vi "Find All Uses.Bundlers.vi"(9 "Fully Qualified Array":string[](array[string]), 10 "dotted name":cluster{"dotted name":string[]}, 11 "VIs":refnum<vi>[](array[refnum])) -> (2 "bundle":refnum<vi>[](array[refnum]), 3 "named bundle":refnum<vi>[](array[refnum]))   [LabVIEW 2020]
uses:
  <vilib>/Utility/traverseref.llb/TRef TravTarget.ctl
  <vilib>/Utility/traverseref.llb/VI Scripting - Traverse.lvlib
  <vilib>/Utility/Data Type/NI_Data Type.lvlib
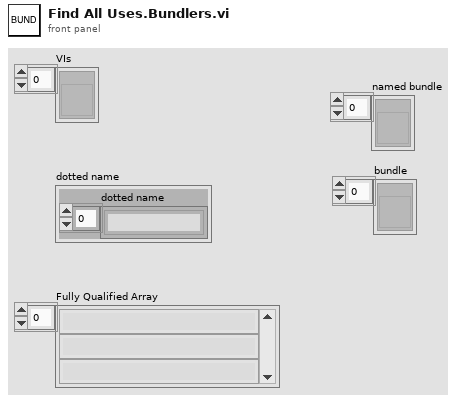
[diagram p1: front panel]
types:
  T1 = typedef "TRef TravTarget.ctl" = enum16{"FP", "BD", "Other"}
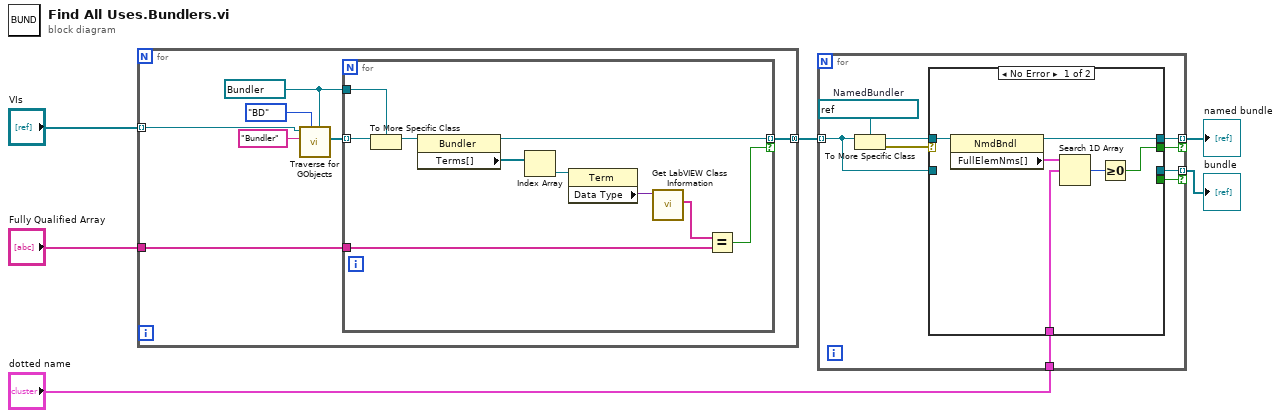
[diagram p0: block diagram]
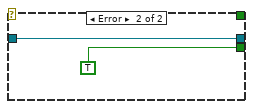
[diagram p2: hidden frame]
diagram:
  n1 = for {
    tunnel: "VIs" -> [w13] mode=indexing
    tunnel: [w8] -> w4 mode=concatenating
    tunnel: "Fully Qualified Array" -> [w7]
    w9 = refnum<vi> refnum ("Other Refnum")
    n2 = call <vilib>:"Traverse for GObjects.vi"("Other Refnum"=w9, "Traverse Target"=TRef_TravTarget."BD", "Class Name"="Bundler", "VI Refnum"=w13) -> ("References"=w10:refnum<vi>[])  [unwired: 4 in, 3 out]
    n3 = for {
      tunnel: w10 -> [w23] mode=indexing
      tunnel: w9 -> [w22]
      tunnel: [w20] -> w8 mode=indexing if=w14
      tunnel: w7 -> [w15]
      n4 = To More Specific Class(target class=w22, reference=w23) -> (specific class reference=w21:refnum<vi>)  [unwired: 1 in, 1 out]
      n5 = property class="Bundler"(reference=w21) -> (reference out=w20:refnum<vi>, "Terms[]"=w19:refnum<vi>[])  [unwired: 1 in, 1 out]
      n6 = Index Array(array=w19) -> (element=w18:refnum<vi>)  [unwired: 1 in]
      n7 = property class="Term"(reference=w18) -> ("Data Type"=w17:variant)  [unwired: 1 in, 2 out]
      n8 = call <vilib>:"Get LabVIEW Class Information.vi"("variant"=w17) -> ("qualified LabVIEW class name"=w16:string[])  [unwired: 8 in, 2 out]
      n9 = Equal?(x=w16, y=w15) -> (x = y?=w14:bool)
    }
  }
  n10 = for {
    tunnel: w4 -> [w29] mode=indexing
    tunnel: [w28] -> w2 mode=indexing if=w27
    tunnel: [w26] -> w3 mode=indexing if=w25
    tunnel: "dotted name" -> [w24]
    w32 = refnum<vi> refnum  # NamedBundler
    n11 = To More Specific Class(target class=w32, reference=w29) -> (specific class reference=w30:refnum<vi>, error out=w31:errorcluster)  [unwired: 1 in]
    n12 = case shown="No Error" w31 {
      tunnel: w30 -> [w36 _]
      tunnel: w29 -> [_ w40]
      tunnel: [_ w40] -> w28
      tunnel: [_ TRUE] -> w27
      tunnel: [w35 _] -> w26
      tunnel: [w34 _] -> w25
      tunnel: w24 -> [w33 _]
      frame No Error {
        n13 = property class="NmdBndl"(reference=w36) -> (reference out=w35:refnum<vi>, "FullElemNms[]"=w38:cluster{string[]}[])  [unwired: 1 in, 1 out]
        n14 = Search 1D Array(1D array=w38, element=w33) -> (index of element=w37:i32)  [unwired: 1 in]
        n15 = Greater Or Equal To 0?(x=w37) -> (x >= 0?=w34:bool)
      }
      frame Error {
      }
    }
  }
  "named bundle" <- w3
  "bundle" <- w2
